vi "Revision Query Core.vi"(8 "error in (no error)":errorcluster, 11 "KIT-QVA in":refnum<class "KIT-QVA.lvclass">) -> (0 "error out":errorcluster, 1 "Firmware Revision":string, 2 "Driver Revision":string, 3 "KIT-QVA out":refnum<class "KIT-QVA.lvclass">)   [LabVIEW 2016, in "KIT-QVA.lvlib" / "KIT-QVA.lvclass"]
doc: "Acestro class imnplementation returning N/A as default for Driver and Firmware Revisions."
uses:
  KIT-QVA.lvclass
  KIT-QVA.lvclass/KIT-QVA.ctl
  CSPP_Core/Actors/CS++DeviceActor/CS++DeviceActor.lvclass
  instr.lib/KIT-QV/KIT QV.lvlib
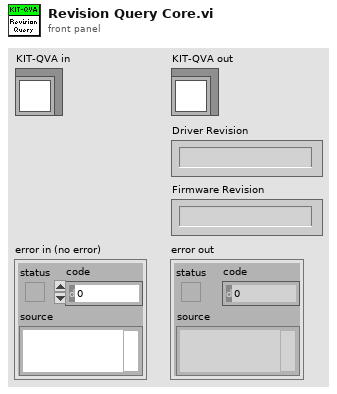
[diagram p1: front panel]
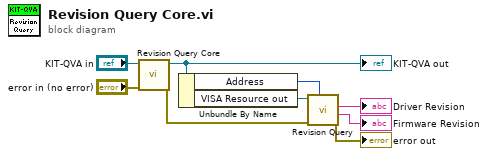
[diagram p0: block diagram]
diagram:
  n1 = call-parent "Revision Query Core.vi"("error in (no error)"="error in (no error)", "CS++DeviceActor in"="KIT-QVA in") -> ("error out"=w7:errorcluster, "CS++DeviceActor out"=w6:refnum<class "KIT-QVA.lvclass">)  [unwired: 6 in, 2 out]
  "KIT-QVA out" <- w6
  n2 = Unbundle By Name(w6) -> ("Address"=w4:u16, "VISA Resource out"=w5:refnum<visa-resource-name>)
  n3 = call "Revision Query.vi"("Address"=w4, "Error In"=w7, "VISA Resource in"=w5) -> ("Error Out"=→"error out":errorcluster, "Instrument Firmware Revision"=→"Firmware Revision":string, "Instrument Driver Revision"=→"Driver Revision":string)  [unwired: 5 in, 1 out]
